vi "未命名 1.vi"() -> ()   [LabVIEW 2017]
panel:
  out "数据值":variant[](array[variant])
  in  "控件索引":i32[](array[numeric])
  in  "字符串":string
  in  "数值 2":i32
  in  "数值":dbl
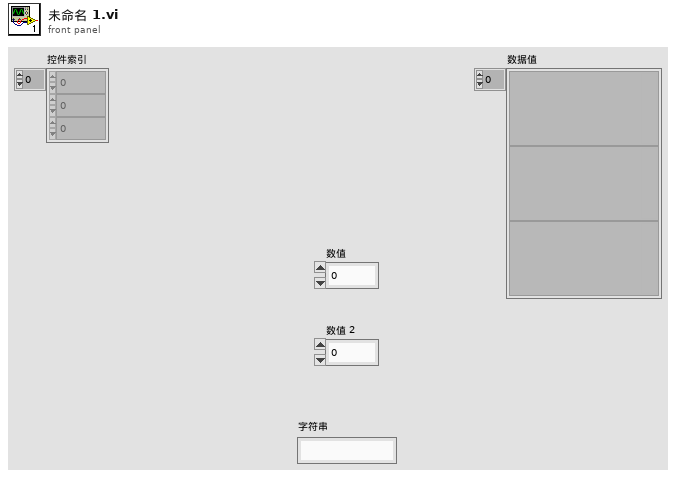
[diagram p1: front panel]
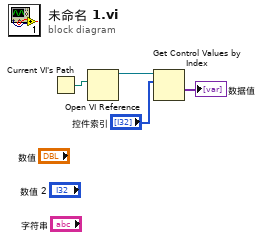
[diagram p0: block diagram]
diagram:
  n1 = Current VI's Path() -> (path=w3:path)
  n2 = Open VI Reference(vi path=w3) -> (vi reference=w4:refnum<vi>)  [unwired: 5 in, 1 out]
  n3 = Get Control Values by Index(0:w4, 1:"控件索引") -> (10:→"数据值":variant[])  [unwired: 1 in, 1 out]
